vi "S2C_VLFT10_Proc_LookupValue.vi"(8 "Error In":errorcluster, 10 "Clear?":bool, 11 "VarName":string) -> (0 "Error Out":errorcluster, 2 "Found?":bool, 3 "VarValue":string)   [LabVIEW 2015]
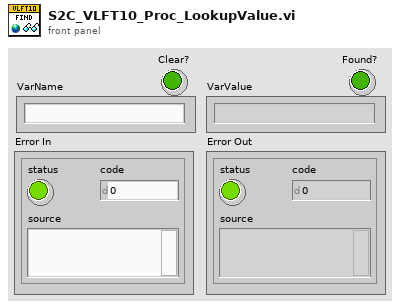
[diagram p1: front panel]
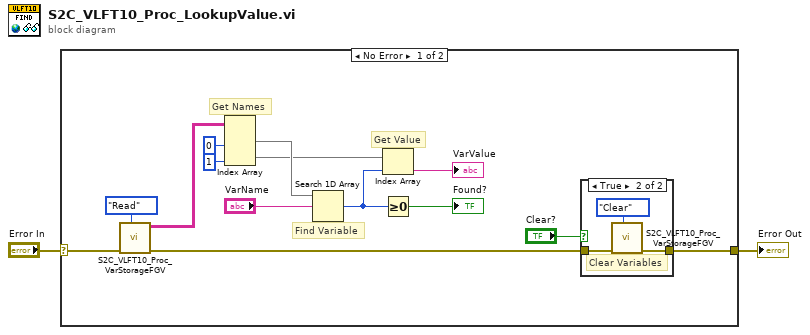
[diagram p0: block diagram]
diagram:
  n1 = case shown="No Error" "Error In" {
    selector: "Error In" -> [w16 w21]
    tunnel: [w4 w21] -> w1
    frame No Error {
      # "Get Value"
      # "Find Variable"
      # "Get Names"
      n2 = call "S2C_VLFT10_Proc_VarStorageFGV.vi"("Action"=enum16{"Read", "Write", "Clear"}."Read", "Error In"=w16) -> ("Error Out"=w5:errorcluster, "Data Out"=w14:string[][])  [unwired: 8 in]
      n3 = Index Array(array=w14, index (col) #1=0 ("disabled index (col)"), index (col) #2=1 ("index (col)")) -> (element #1=w12:string[], element #2=w9:string[])  [unwired: 2 in]
      n4 = Search 1D Array(1D array=w12, element="VarName") -> (index of element=w7:i32)  [unwired: 1 in]
      n5 = Index Array(array=w9, index=w7) -> (element=→"VarValue":string)
      n6 = Greater Or Equal To 0?(x=w7) -> (x >= 0?=→"Found?":bool)
      n7 = case shown="True" "Clear?" {
        tunnel: w5 -> [w17 w19]
        tunnel: [w17 w18] -> w4
        frame False {
        }
        frame True {
          # "Clear Variables"
          n8 = call "S2C_VLFT10_Proc_VarStorageFGV.vi"("Action"=enum16{"Read", "Write", "Clear"}."Clear", "Error In"=w19) -> ("Error Out"=w18:errorcluster)  [unwired: 8 in, 1 out]
        }
      }
    }
    frame Error {
    }
  }
  "Error Out" <- w1
